vi "Done Face.vi"(8 "error in (no error)":errorcluster, 11 "face in":i64) -> (0 "error out":errorcluster)   [LabVIEW 2023, in "Freetype Drawer.lvlib"]
uses:
  Freetype Drawer.lvlib
  libfreetype.dll
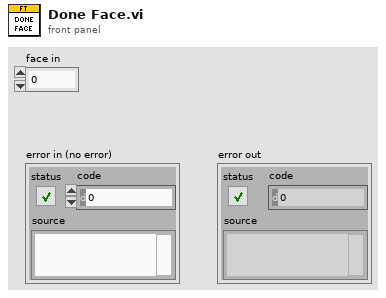
[diagram p1: front panel]
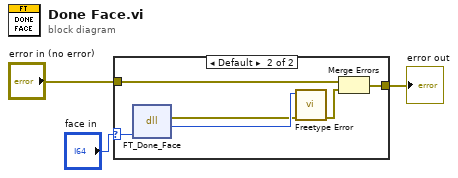
[diagram p0: block diagram]
diagram:
  n1 = case shown="Default" "face in" {
    selector: "face in" -> [_ w10]
    tunnel: "error in (no error)" -> [w4 w9]
    tunnel: [w4 w8] -> w1
    frame 0 {
    }
    frame Default {
      n2 = dll-call lib="E:/Labview/LV 2023/Libs/LV Symbol/Freetype Drawer/Wrappers/libfreetype.dll" fn="FT_Done_Face"("face"=w10) -> (error out=w6:errorcluster, "error"=w7:i32)  [unwired: 4 in, 1 out]
      n3 = call "Freetype Error.vi"("error in (no error)"=w6, "Error"=w7) -> ("error out"=w5:errorcluster)  [unwired: 9 in]
      n4 = Merge Errors(w9, w5) -> (w8:errorcluster)
    }
  }
  "error out" <- w1
